vi "Read Trace.vi"(8 "error in (no error)":errorcluster, 9 "Maximum Time (10000 ms)":i32=10000, 10 "Trace Name (1: Trace 1)":u16(ring)=1 items=["Trace 1"=1, "Trace 2"=2, "Trace 3"=3], 11 "VISA resource name":refnum<visa-resource-name>) -> (0 "error out":errorcluster, 2 "Trace Waveform":T1(graph), 3 "VISA resource name out":refnum<visa-resource-name>)   [LabVIEW 2014, in "Agilent ESA PSA Series.lvlib"]
doc: "Reads a trace from the spectrum analyzer."
uses:
  Agilent ESA PSA Series.lvlib
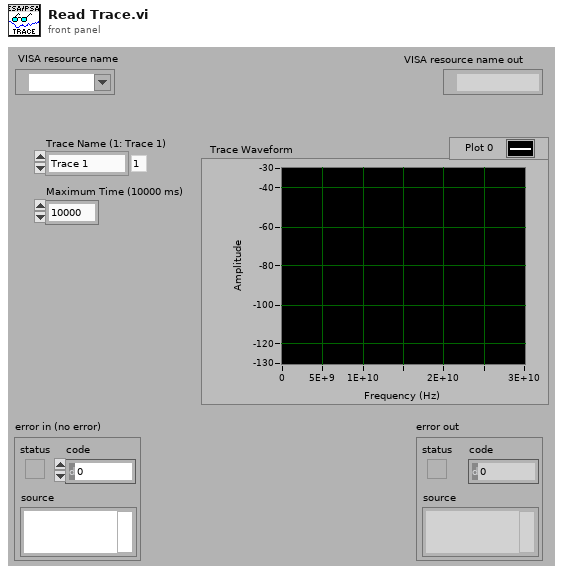
[diagram p1: front panel]
types:
  T1 = cluster{"Initial X":dbl, "X Increment":dbl, "Trace Array":dbl[]}
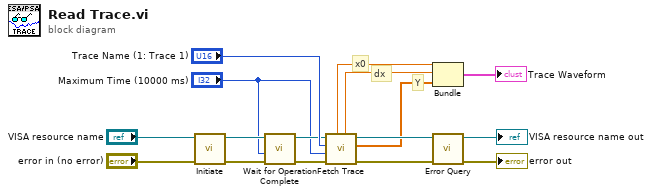
[diagram p0: block diagram]
diagram:
  # "Y"
  # "dx"
  # "x0"
  n1 = call "Initiate.vi"("error in (no error)"="error in (no error)", "VISA resource name"="VISA resource name") -> ("error out"=w4:errorcluster, "VISA resource name out"=w5:refnum<visa-resource-name>)  [unwired: 8 in]
  n2 = call "Wait for Operation Complete.vi"("error in (no error)"=w4, "Maximum Time (10000ms)"="Maximum Time (10000 ms)", "VISA resource name"=w5) -> ("error out"=w2:errorcluster, "VISA resource name out"=w3:refnum<visa-resource-name>)  [unwired: 7 in]
  n3 = call "Fetch Trace.vi"("error in (no error)"=w2, "Timeout (10000 ms)"="Maximum Time (10000 ms)", "Trace Name (1: Trace 1)"="Trace Name (1: Trace 1)", "VISA resource name"=w3) -> ("error out"=w14:errorcluster, "Trace Array"=w9:dbl[], "VISA resource name out"=w16:refnum<visa-resource-name>, "X Increment"=w12:dbl, "Initial X"=w11:dbl)  [unwired: 3 in]
  n4 = Bundle("Initial X"=w11, "X Increment"=w12, "Trace Array"=w9) -> (→"Trace Waveform":T1)  [unwired: 1 in]
  n5 = call "Error Query.vi"("error in (no error)"=w14, "VISA resource name"=w16) -> ("error out"=→"error out":errorcluster, "VISA resource name out"=→"VISA resource name out":refnum<visa-resource-name>)  [unwired: 6 in, 2 out]
